vi "newSubvi MultiROI Image.vi"(2 "ROISelected":u32, 4 "Snap":bool, 5 "ImageRepeatNum":u32, 6 "ROIListBoxIn":string[][](array[string]), 7 "BaseFileName":string) -> (0 "ImagingDone":bool)   [LabVIEW 2012]
uses:
  ProSCI Global.vi
panel:
  out "TileSuffix":string[](array[string])
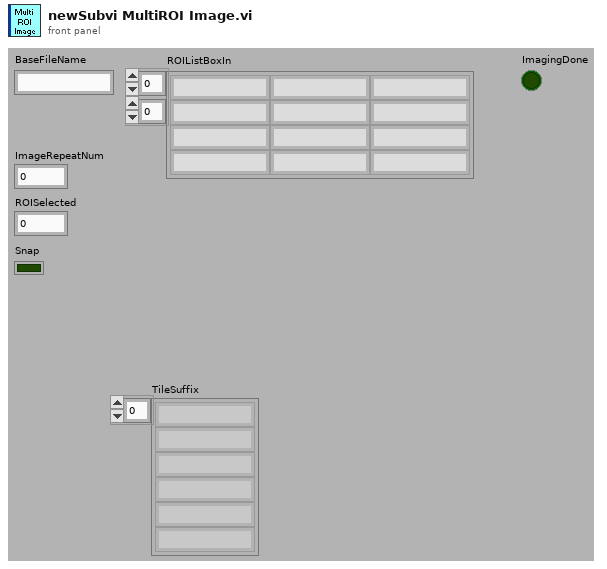
[diagram p1: front panel]
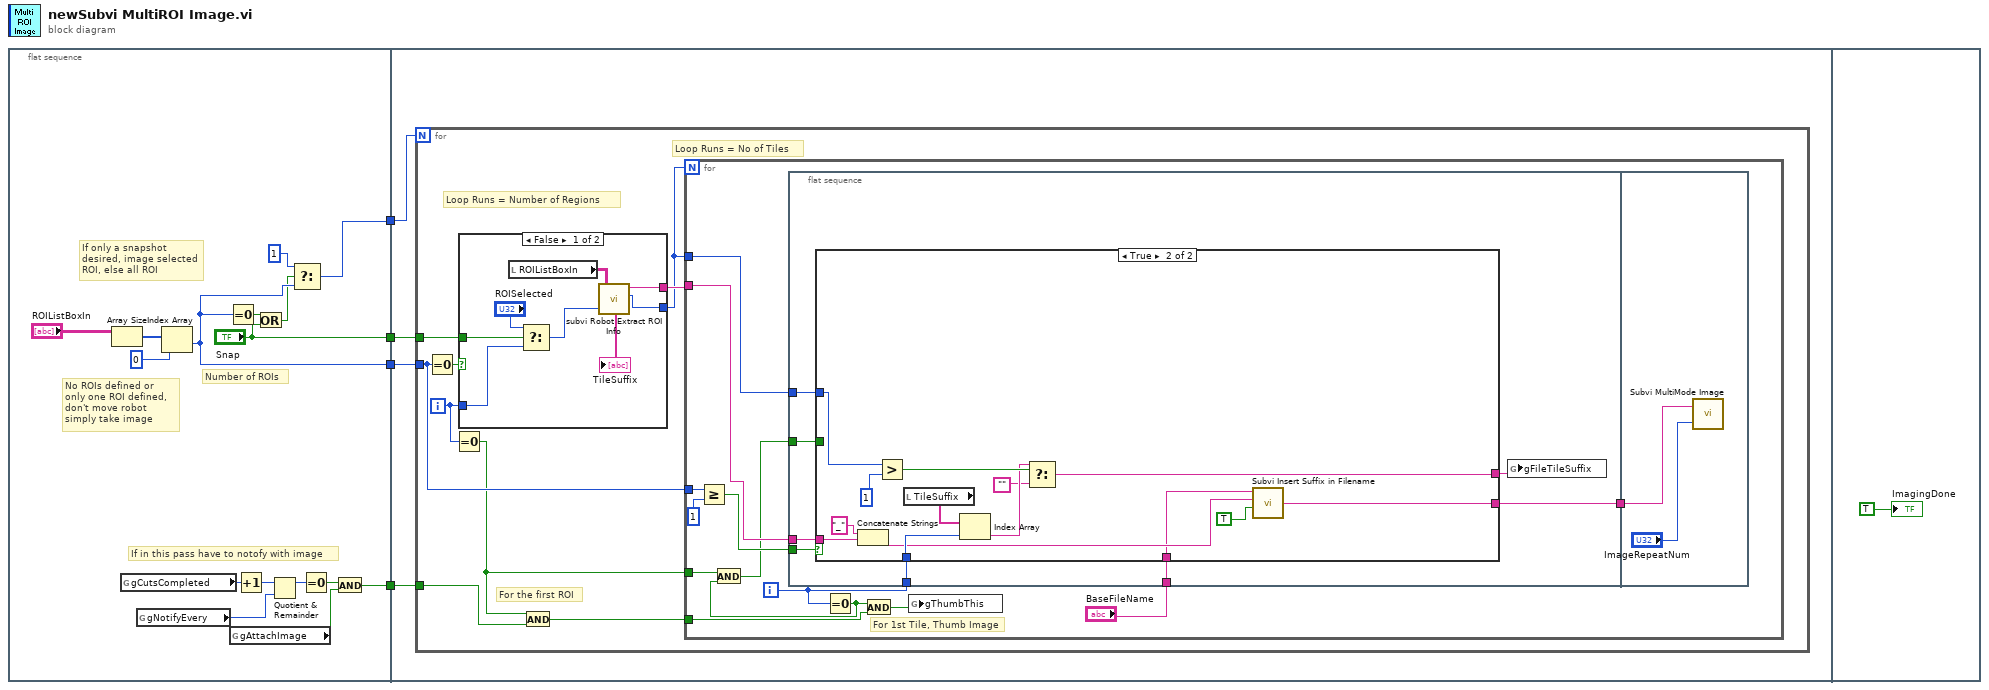
[diagram p0: block diagram]
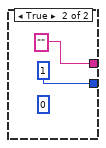
[diagram p2: hidden frame]
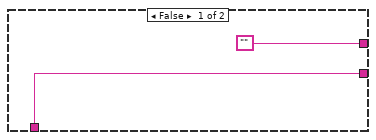
[diagram p3: hidden frame]
diagram:
  n1 = flat-sequence {
    tunnel: [w16] -> w4
    tunnel: ["Snap"] -> w3
    tunnel: [w14] -> w2
    tunnel: [w5] -> w1
    tunnel: w4 -> [w24]
    tunnel: w3 -> [w23]
    tunnel: w2 -> [w22]
    tunnel: w1 -> [w21]
    frame #0 {
      # "If in this pass have to notofy with image"
      # "If only a snapshot\ndesired, image selected\nROI, else all ROI"
      # "No ROIs defined or\nonly one ROI defined,\ndon't move robot\nsimply take image"
      # "Number of ROIs"
      n2 = Array Size(array="ROIListBoxIn") -> (size(s)=w20:i32[])
      n3 = global read "ProSCI Global.vi" "gCutsCompleted"() -> (w11:i32)
      n4 = global read "ProSCI Global.vi" "gNotifyEvery"() -> (w9:u32)
      n5 = Index Array(array=w20, index=0) -> (element=w14:i32)
      n6 = Equal To 0?(x=w14) -> (x = 0?=w13:bool)
      n7 = global read "ProSCI Global.vi" "gAttachImage"() -> (w6:bool)
      n8 = Increment(x=w11) -> (x+1=w10:i32)
      n9 = Or(x=w13, y="Snap") -> (x .or. y?=w12:bool)
      n10 = Quotient & Remainder(x=w10, y=w9) -> (x-y*floor(x/y)=w8:u32)  [unwired: 1 out]
      n11 = Select(t=1, s=w12, f=w14) -> (s? t:f=w16:i32)
      n12 = Equal To 0?(x=w8) -> (x = 0?=w7:bool)
      n13 = And(x=w7, y=w6) -> (x .and. y?=w5:bool)
    }
    frame #1 {
      n14 = for {
        N: w24 -> [_]
        tunnel: w23 -> [w32]
        tunnel: w22 -> [w30]
        tunnel: w21 -> [w27]
        i -> [w28]
        # "For the first ROI"
        # "Loop Runs = No of Tiles"
        # "Loop Runs = Number of Regions"
        n15 = Equal To 0?(x=w30) -> (x = 0?=w31:bool)
        n16 = Equal To 0?(x=w28) -> (x = 0?=w25:bool)
        n17 = case shown="False" w31 {
          tunnel: [w41 u32 1 ("TotalTiles")] -> w29
          tunnel: [w40 "" ("ROIName")] -> w33
          tunnel: w32 -> [w39 _]
          tunnel: w28 -> [w38 _]
          frame False {
            n18 = local read "ROIListBoxIn"() -> (w37:string[][])
            n19 = Select(t="ROISelected", s=w39, f=w38) -> (s? t:f=w35:u32)
            n20 = call "subvi Robot Extract ROI Info.vi"("ROIListBoxIn"=w37, "Selection"=w35) -> ("ROIName"=w40:string, "TotalTiles"=w41:u32, "TileSuffix"=→"TileSuffix":string[])  [unwired: 1 out]
          }
          frame True {
            (unwired) u32 0 ("XYListOffset")
          }
        }
        n21 = And(x=w25, y=w27) -> (x .and. y?=w26:bool)
        n22 = for {
          N: w29 -> [_]
          tunnel: w33 -> [w54]
          tunnel: w30 -> [w52]
          tunnel: w29 -> [w53]
          tunnel: w26 -> [w48]
          tunnel: w25 -> [w44]
          i -> [w49]
          # "For 1st Tile, Thumb Image"
          n23 = Greater Or Equal?(x=w52, y=1 ("x")) -> (x >= y?=w55:bool)
          n24 = flat-sequence {
            tunnel: w49 -> [w64]
            tunnel: w55 -> [w63]
            tunnel: w53 -> [w62]
            tunnel: w54 -> [w61]
            tunnel: w45 -> [w60]
            tunnel: "BaseFileName" -> [w59]
            tunnel: [w58] -> w50
            tunnel: w50 -> [w81]
            frame #0 {
              n25 = case shown="True" w63 {
                tunnel: w64 -> [_ w76]
                tunnel: w62 -> [_ w79]
                tunnel: w61 -> [_ w77]
                tunnel: w60 -> [_ _]
                tunnel: w59 -> [w66 w69]
                tunnel: [w66 w68] -> w58
                tunnel: ["" w67] -> w57
                frame False {
                }
                frame True {
                  n26 = Concatenate Strings("_" ("string"), w77) -> (w70:string)
                  n27 = Greater?(x=w79, y=u32 1) -> (0:w74:bool)
                  n28 = local read "TileSuffix"() -> (w75:string[])
                  n29 = Index Array(array=w75, index=w76) -> (element=w73:string)
                  n30 = Select(t=w73, s=w74, f="") -> (s? t:f=w67:string)
                  n31 = call "Subvi Insert Suffix in Filename.vi"("OnlyROI"=TRUE, "Suffix"=w70, "InFileName"=w69) -> ("OutFileName"=w68:string)  [unwired: 1 in]
                }
              }
              n32 = global write "ProSCI Global.vi" "gFileTileSuffix"(w57) -> ()
            }
            frame #1 {
              n33 = call "Subvi MultiMode Image.vi"("ImageRepeatNum"="ImageRepeatNum", "InFileName"=w81) -> ()  [unwired: 2 out]
            }
          }
          n34 = Equal To 0?(x=w49) -> (x = 0?=w46:bool)
          n35 = And(x=w44, y=w46) -> (x .and. y?=w45:bool)
          n36 = And(x=w46, y=w48) -> (x .and. y?=w47:bool)
          n37 = global write "ProSCI Global.vi" "gThumbThis"(w47) -> ()
        }
      }
    }
    frame #2 {
      "ImagingDone" <- TRUE
    }
  }
